vi "split.vi"(8 "error in (no error) 2":errorcluster caption="entrée d'erreur (pas d'erreur)", 9 "In":cluster{"X":dbl[][], "y":dbl[], "groups":dbl[]}={"X"=[[1.0, 2.0], [3.0, 4.0], [5.0, 6.0], [7.0, 8.0]], "y"=[1.0, 2.0, 3.0, 4.0], "groups"=[]}, 10 "n_splits":u8=2, 11 "Splitter en entrée":refnum<class "Splitter.lvclass">) -> (0 "error out 2":errorcluster caption="sortie d'erreur", 2 "Out":T1={"train_index"=[[1.0, 2.0], [3.0, 4.0], [5.0, 6.0], [7.0, 8.0]], "test_index"=[[1.0, 2.0], [3.0, 4.0], [5.0, 6.0], [7.0, 8.0]]}, 3 "Splitter en sortie":refnum<class "Splitter.lvclass">)   [LabVIEW 2020, in "Splitter.lvclass"]
uses:
  Splitter.lvclass
  Splitter.lvclass/Splitter.ctl
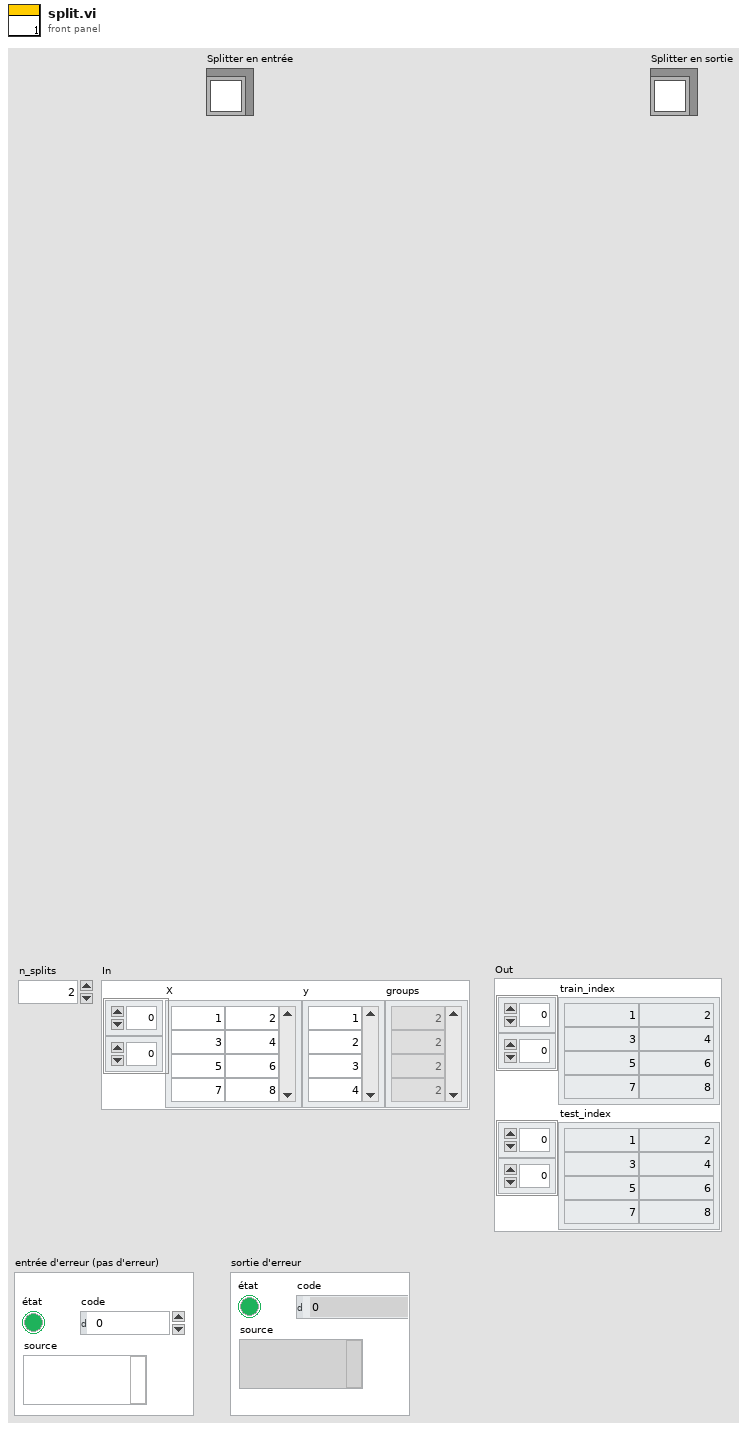
[diagram p1: front panel]
types:
  T1 = cluster{"train_index":dbl[][], "test_index":dbl[][]}
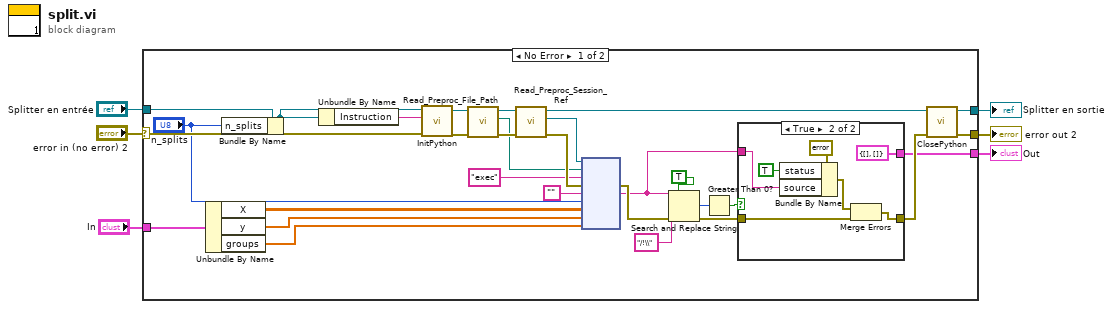
[diagram p0: block diagram]
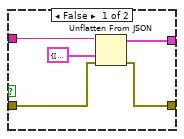
[diagram p2: hidden frame]
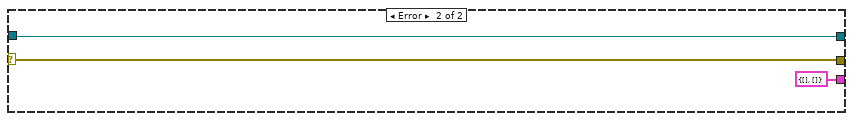
[diagram p3: hidden frame]
diagram:
  n1 = case shown="No Error" "error in (no error) 2" {
    selector: "error in (no error) 2" -> [w36 w50]
    tunnel: [w13 w51] -> w5
    tunnel: "Splitter en entrée" -> [w33 w51]
    tunnel: [w35 w50] -> w3
    tunnel: "In" -> [w11 _]
    tunnel: [w7 T1 {"train_index"=[], "test_index"=[]} ("Cluster")] -> w1
    frame No Error {
      n2 = Unbundle By Name(w11) -> ("X"=w10:dbl[][], "y"=w9:dbl[], "groups"=w8:dbl[])
      n3 = Bundle By Name(cluster=w33, "n_splits"="n_splits") -> (w18:refnum<class "Splitter.lvclass">)
      n4 = Unbundle By Name(w18) -> ("Instruction"=w34:string)
      n5 = call-dynamic "InitPython.vi"("error in (no error)"=w36, "Python Instruction"=w34, "Scikit-learn en entrée"=w18) -> ("error out"=w16:errorcluster, "Scikit-learn en sortie"=w17:refnum<class "Splitter.lvclass">)  [unwired: 7 in]
      n6 = call-dynamic "Read_Preproc_File_Path.vi"("error in (no error)"=w16, "Python in"=w17) -> ("error out"=w31:errorcluster, "File_Path"=w29:path, "Python out"=w30:refnum<class "Splitter.lvclass">)  [unwired: 7 in]
      n7 = call-dynamic "Read_Preproc_Session_Ref.vi"("error in (no error)"=w31, "Python in"=w30) -> ("error out"=w32:errorcluster, "Session_ref"=w28:refnum<k35>, "Python out"=w14:refnum<class "Splitter.lvclass">)  [unwired: 7 in]
      n8 = node(w28, w29, "exec" ("function name"), w32, "", "n_splits", w10, w9, w8) -> (w27:errorcluster, w26:string)  [unwired: 4 in, 3 out]
      n9 = Search and Replace String(replace all?=TRUE ("replace all? (F)"), input string=w26, search string="/!\\", error in=w27) -> (number of replacements=w24:i32, error out=w23:errorcluster)  [unwired: 4 in, 2 out]
      n10 = Greater Than 0?(x=w24) -> (x > 0?=w25:bool)
      n11 = case shown="True" w25 {
        tunnel: w23 -> [w38 w45]
        tunnel: [w37 w44] -> w15
        tunnel: w26 -> [w39 w43]
        tunnel: [w40 T1 {"train_index"=[], "test_index"=[]} ("Cluster")] -> w7
        frame False {
          n12 = Unflatten From JSON(JSON string=w39, type and defaults=T1 {"train_index"=[[1.0, 2.0], [3.0, 4.0], [5.0, 6.0], [7.0, 8.0]], "test_index"=[[1.0, 2.0], [3.0, 4.0], [5.0, 6.0], [7.0, 8.0]]} ("Cluster"), error in (no error)=w38) -> (value=w40:T1, error out=w37:errorcluster)  [unwired: 4 in]
        }
        frame True {
          n13 = Bundle By Name(cluster=errorcluster {"status"=FALSE, "code"=0, "source"=""} ("error constant"), "status"=TRUE, "source"=w43) -> (w46:errorcluster)
          n14 = Merge Errors(w46, w45) -> (w44:errorcluster)
        }
      }
      n15 = call-dynamic "ClosePython.vi"("error in (no error)"=w15, "Scikit-learn en entrée"=w14) -> ("error out"=w35:errorcluster, "Scikit-learn en sortie"=w13:refnum<class "Splitter.lvclass">)  [unwired: 8 in]
    }
    frame Error {
    }
  }
  "Splitter en sortie" <- w5
  "error out 2" <- w3
  "Out" <- w1
